vi "WTR.vi"(0 "System no.":i32=1 min=1 max=4 step=1, 2 "Generator ID":i32[](array[numeric]) min=0 step=1, 3 "Table rate":i32[](array[numeric]) min=1 step=1, 4 "Interpolation type":i32[](array[numeric]) min=0 step=1, 5 "error in":errorcluster) -> (19 "error out":errorcluster)   [LabVIEW 2020]
doc: "Set wave generator table rate. This VI will change the sampling interval of the wave generator. When Generator ID is zero all generators are selected, otherwise each generator is selected individually. Table Rate sets the duration of the wave table points as a multiple of the servo interval time. When a Table rate higher than 1 is set, Interpolation type can be used to join each wave table point by an interpolation.\n\nC-413 : The following Interpolation types can be selected:\n0 = no interpolation\nGenerator ID must be 0 because values can only be set for all generators.\n\nC-886: The following Interpolation types can be selected:\n0 = no interpolation, 1 = straight line \nTable rate values and Interpolation type for any Generator ID are valid for all wave generators (cannot be set differently). \n\nC-887: The following Interpolation types can be selected:\n0 = no interpolation, 1 = straight line \nTable rate values and Interpolation type for any Generator ID are valid for all wave generators (cannot be set differently). \n\nC-891: The following Interpolation types can be selected:\n0 = no interpolation, 1 = straight line.\nGenerator ID can be 0 or 1 as there is only one generator.\n\nE-517, E-518: Interpolation type must be 0. Generator ID can be 1 to 3. WTR sets the value of the Wave Generator Table Rate parameter, ID 0x13000109, in volatile memory. You can set the wave table rate also using the CFG wave type (see WAV command) or by directly changing the parameter with SPA.\n\nE-709: The following Interpolation types can be selected:\n0 = no interpolation \nGenerator ID can be 0 or 1 as there is only one generator.\n\nE-712: The following Interpolation types can be selected:\n0 = no interpolation, 1 = straight line\nGenerator ID must be 0 because values can only be set for all generators.\n\nE-725, E-727: The following Interpolation types can be selected:\n0 = no interpolation, 1 = straight line\nGenerator ID must be 0 because values can only be set for all generators.\n\nE-753: The following Interpolation types can be selected:\n0 = no interpolation, 1 = straight line. Generator ID must be 0 because values can only be set for all generators.\n\nE-754: The following Interpolation types can be selected:\n0 = no interpolation, 1 = straight line. Generator ID must be 0 because values can only be set for all generators."
panel:
  # "Set Wave Generator Table Rate."
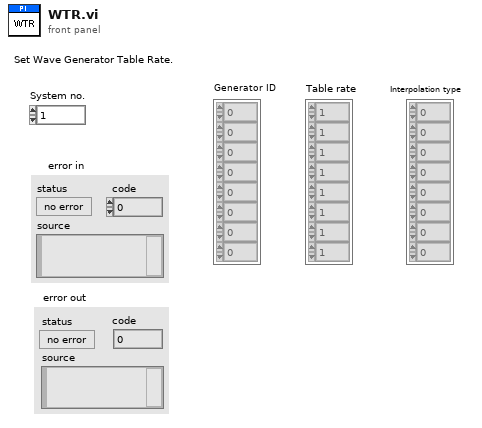
[diagram p1: front panel]
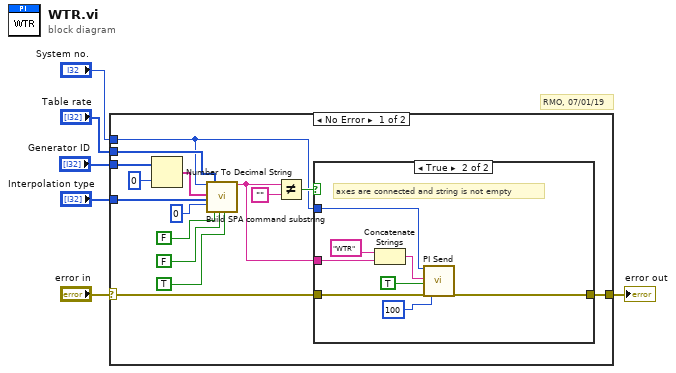
[diagram p0: block diagram]
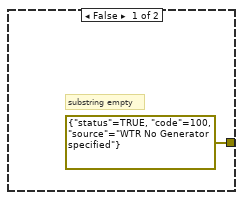
[diagram p2: hidden frame]
diagram:
  # "RMO, 07/01/19"
  n1 = case shown="No Error" "error in" {
    selector: "error in" -> [w7 w31]
    tunnel: [w21 w31] -> w6
    tunnel: "System no." -> [w16 _]
    tunnel: "Generator ID" -> [w11 _]
    tunnel: "Table rate" -> [w18 _]
    tunnel: "Interpolation type" -> [w8 _]
    frame No Error {
      n2 = Number To Decimal String(number=w11, width (-)=i16 0) -> (decimal integer string=w10:string[])
      n3 = call "Build SPA command substring.vi"("System no."=w16, "Axes to set"=w10, "Parameter values"=w8, "No. of digits"=i16 0, "Parameter number"=w18, "Parameter no. format \n(Decimal: FALSE)"=FALSE ("Parameter no. format \n(Decimal: FALSE)"), "Parameter format \n(Num.: FALSE)"=FALSE ("Parameter format \n(Num.: FALSE)"), "With space?"=TRUE) -> ("SPA command substring"=w19:string)  [unwired: 2 in, 9 out]
      n4 = Not Equal?(x=w19, y="") -> (x != y?=w17:bool)
      n5 = case shown="True" w17 {
        tunnel: w19 -> [_ w29]
        tunnel: [errorcluster {"status"=TRUE, "code"=100, "source"="WTR No Generator specified"} ("error out") w23] -> w21
        tunnel: w7 -> [_ w26]
        tunnel: w16 -> [_ w25]
        frame False {
          # "substring empty"
        }
        frame True {
          # "axes are connected and string is not empty"
          n6 = Concatenate Strings("WTR", w29) -> (w27:string)
          n7 = call "PI Send.vi"("System no."=w25, "String to send"=w27, "Attach termination char.?"=TRUE ("Attach Linefeed?"), "error in"=w26, "Delay before error check (ms)"=u32 100 ("milliseconds to wait")) -> ("error out"=w23:errorcluster)  [unwired: 1 in, 13 out]
        }
      }
    }
    frame Error {
    }
  }
  "error out" <- w6
